vi "sub shift_leds.vi"(3 "error out":errorcluster, 5 "output array 2":u8[](array[numeric])) -> (0 "error out 2":errorcluster, 1 "string":string, 2 "return count":u32, 4 "VISA resource name out":refnum<visa-resource-name>)   [LabVIEW 2016]
panel:
  out "string 2":string
  in  "output array":u8[](array[numeric])
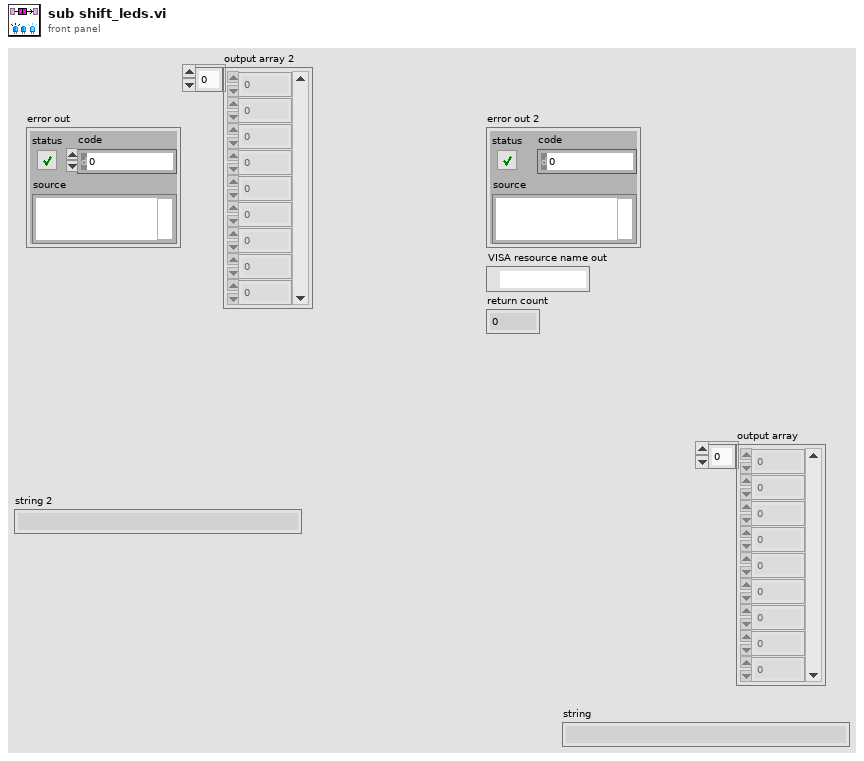
[diagram p1: front panel]
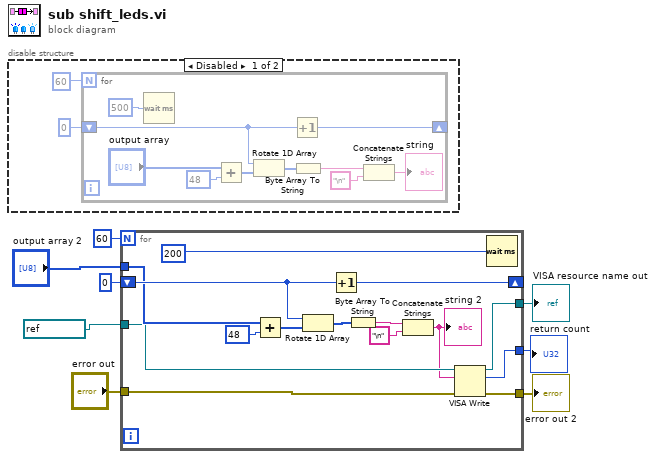
[diagram p0: block diagram]
diagram:
  n1 = disable-structure shown="Disabled" {
    frame Disabled {
      n2 = for {
        N: 60 -> [_]
        shift-right: [w17] -> _
        shift-left: 0 ("n") -> [w18]
        n3 = Wait (ms)(milliseconds to wait=u32 500) -> ()  [unwired: 1 out]
        n4 = Add(x="output array", y=48) -> (x+y=w12:i32[])
        n5 = Rotate 1D Array(1:w12, 2:w18) -> (0:w19:i32[])
        n6 = Increment(x=w18) -> (x+1=w17:i32)
        n7 = Byte Array To String(unsigned byte array=w19) -> (string=w15:string)
        n8 = Concatenate Strings(w15, "\n") -> (→"string":string)
      }
    }
    frame Enabled {
    }
  }
  n9 = for {
    N: 60 -> [_]
    shift-right: [w32] -> _
    shift-left: u8 0 -> [w33]
    tunnel: "output array 2" -> [w27]
    tunnel: refnum<visa-resource-name> "COM5" ("VISA resource name out") -> [w26]
    tunnel: "error out" -> [w25]
    tunnel: [w23] -> w3
    tunnel: [w22] -> w4
    tunnel: [w21] -> w2
    n10 = Add(x=w27, y=48) -> (x+y=w28:i32[])
    n11 = Rotate 1D Array(1:w28, 2:w33) -> (0:w34:i32[])
    n12 = Increment(x=w33) -> (x+1=w32:u8)
    n13 = Byte Array To String(unsigned byte array=w34) -> (string=w30:string)
    n14 = Concatenate Strings(w30, "\n") -> (w24:string)
    "string 2" <- w24
    n15 = VISA Write(VISA resource name=w26, write buffer=w24, error in (no error)=w25) -> (VISA resource name out=w23:refnum<visa-resource-name>, return count=w21:u32, error out=w22:errorcluster)
    n16 = Wait (ms)(milliseconds to wait=u32 200) -> ()  [unwired: 1 out]
  }
  "error out 2" <- w4
  "VISA resource name out" <- w3
  "return count" <- w2
